vi "Motic Get Offset Range.vi"(8 "error in (no error)":errorcluster, 11 "camera":i32) -> (0 "error out":errorcluster, 1 "min out":i32, 2 "max out":i32, 3 "camera out":i32)   [LabVIEW 2012, in "MoticApi.lvlib"]
doc: "MOTICAPI bool Motic_GetOffsetRange(MUCam_Handle camera, int *min, int *max);"
uses:
  MoticApi.lvlib
  MoticApi.dll
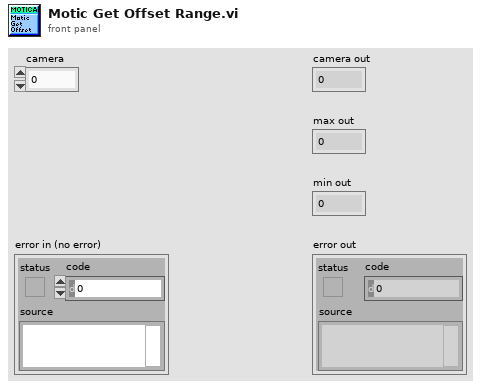
[diagram p1: front panel]
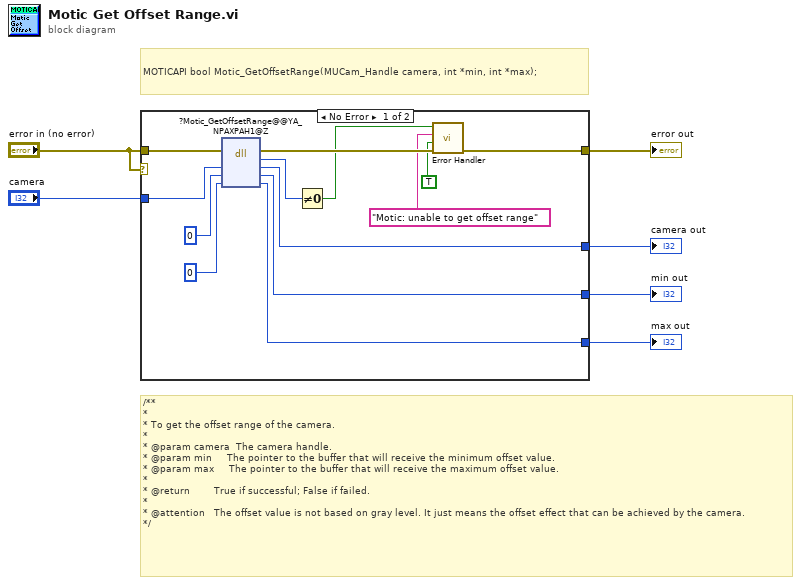
[diagram p0: block diagram]
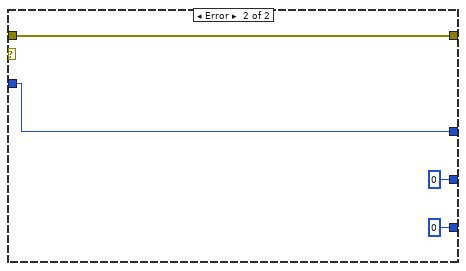
[diagram p2: hidden frame]
diagram:
  # "/**\n*\n* To get the offset range of the camera.\n*\n* @param camera  The camera handle.\n* @param min     The pointer to the buffer that will receive the minimum offset value.\n* @param max     The pointer to the buffer that will receive the maximum offset value.\n*\n* @return        True if successful; False if failed.\n*\n* @attention   The offset value is not based on gray level. It just means the offset effect that can be achieved by the camera.\n*/"
  # "MOTICAPI bool Motic_GetOffsetRange(MUCam_Handle camera, int *min, int *max);"
  n1 = case shown="No Error" "error in (no error)" {
    tunnel: "camera" -> [w18 w22]
    tunnel: [w17 w22] -> w5
    tunnel: [w15 0 ("min")] -> w4
    tunnel: [w14 0 ("max")] -> w3
    tunnel: "error in (no error)" -> [w13 w23]
    tunnel: [w12 w23] -> w2
    frame No Error {
      n2 = dll-call lib="C:/Users/TTS-Digital/Desktop/MoticApi/MoticApi_git/MoticApi/MoticApi.*" fn="?Motic_GetOffsetRange@@YA_NPAXPAH1@Z"(error in=w13, "camera"=w18, "min"=0, "max"=0 ("min")) -> (error out=w11:errorcluster, "return type"=w19:u8, "camera"=w17:i32, "min"=w15:i32, "max"=w14:i32)  [unwired: 2 in, 1 out]
      n3 = Not Equal To 0?(x=w19) -> (x != 0?=w10:bool)
      n4 = call "Error Handler.vi"("error in (no error)"=w11, "Is warning?"=TRUE, "Error message"="Motic: unable to get offset range", "Function return"=w10) -> ("error out"=w12:errorcluster)  [unwired: 7 in]
    }
    frame Error {
    }
  }
  "camera out" <- w5
  "min out" <- w4
  "max out" <- w3
  "error out" <- w2
